vi "Process.vi"(8 "error in (no error)":errorcluster, 11 "Slave Test Runner In":refnum<class "Slave Test Runner.lvclass">) -> (0 "error out":errorcluster, 3 "Slave Test Runner Out":refnum<class "Slave Test Runner.lvclass">)   [LabVIEW 2020, in "Slave Test Runner.lvclass"]
uses:
  Slave Test Runner.lvclass
  C:/Users/anton/Documents/GitHub/LUnit/source/Application Framework/Process Classes/Process/Process.lvclass
  Application Framework/Process Classes/Process/Process.lvclass/Process.ctl
  Slave Test Runner.lvclass/Slave Test Runner.ctl
  Test Case/LUnit Test Case.lvclass
  Test Case/LUnit Test Case.lvclass/LUnit Test Case.ctl
  Result Classes/Method Result/Method Result.lvclass/Method Result.ctl
  Result Classes/Test Case Result/Test Case Result.lvclass/Test Case Result.ctl
  Result Collector/Result Collector.lvclass/Result Collector.ctl
  Result Collector/Result Collector.lvclass
  Private/SubVIs/Get all tests.vi
  Test Case/Community/SubVIs/Pre Test Case Reset.vi
  Private/SubVIs/Shuffle Test Methods.vi
  Private/SubVIs/Obtain Semaphores.vi
  Private/SubVIs/Write Test Case object to front panel control.vi
  Test Case/Community/SubVIs/Pre Method Reset.vi
  Test Case/Community/SubVIs/Get Test Method Result.vi
  Test Case/Community/SubVIs/Check For Errors.vi
  Private/SubVIs/Read Test Case object from front panel control.vi
  <vilib>/Utility/error.llb/Clear Errors.vi
  Private/SubVIs/Check Aborted.vi
  Private/SubVIs/Acquire Semaphore.vi
  Private/SubVIs/Release Semaphore.vi
  Private/SubVIs/Wait on VI to Execute.vi
  Test Case/Community/SubVIs/Set Test Method End Time.vi
  Private/SubVIs/Publish Method Result.vi
  Private/SubVIs/Publish Case Result.vi
  Test Case/Public/Accessors/Read Test Case Result.vi
  Application Framework/Process Classes/Process/Public/Accessors/Read Process Name.vi
  Test Case/Public/Accessors/Read Enabled Test Methods.vi
  Test Case/Private/SubVIs/Pre Allocate Method Results.vi
  Private/SubVIs/Shuffle Test Methods.vi/2fc74b80-6deb-4f17-a78e-34401938511c.vi
  Result Classes/Test Case Result/Public/Accessors/Read Method Results.vi
  Result Classes/Test Case Result/Community/Handle Error.vi
  Result Classes/Test Case Result/Community/Set Method End Time.vi
  Result Collector/Public/API/Collect Method Results.vi
  Result Collector/Public/API/Collect Case Result.vi
  Test Case/Private/SubVIs/Read Test Case Name.vi
  Result Classes/Test Case Result/Community/Preallocate Method Results.vi
  Result Classes/Method Result/Public/Read Status.vi
  Result Classes/Method Result/Community/Accessors/Generate Error.vi
  Result Classes/Method Result/Community/Accessors/Write Execution time.vi
  Result Classes/Method Result/Community/Accessors/Write Test Method Name.vi
  Result Classes/Method Result/Community/Accessors/Write Test Case.vi
  <vilib>/Utility/error.llb/Error Cluster From Error Code.vi
  <vilib>/Utility/LVClass/Get LV Class Name.vi
  <vilib>/Utility/semaphor.llb/Obtain Semaphore Reference.vi
  <vilib>/Utility/semaphor.llb/Acquire Semaphore.vi
  <vilib>/Utility/semaphor.llb/Release Semaphore.vi
  <vilib>/Utility/semaphor.llb/Release Semaphore Reference.vi
  Application Framework/Process Classes/Error Handler/Private/SubVIs/Get Error Queue Name.vi
  Result Classes/Test Case Result/Test Case Result.lvclass
  Result Classes/Method Result/Method Result.lvclass
  Application Framework/Process Classes/Process/Process.lvclass
  Application Framework/Process Classes/Error Handler/Error Handler.lvclass
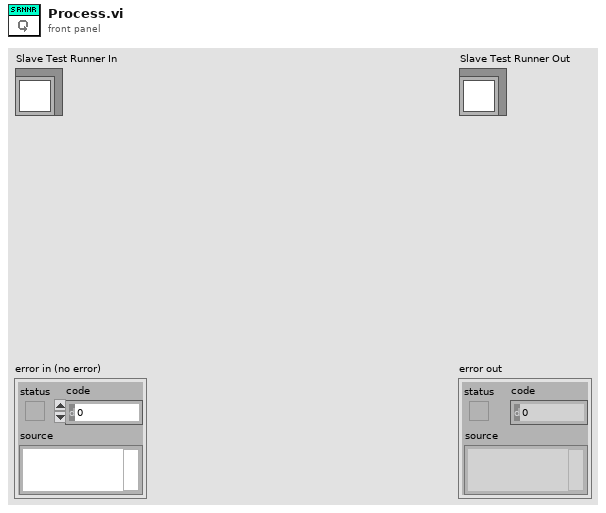
[diagram p1: front panel]
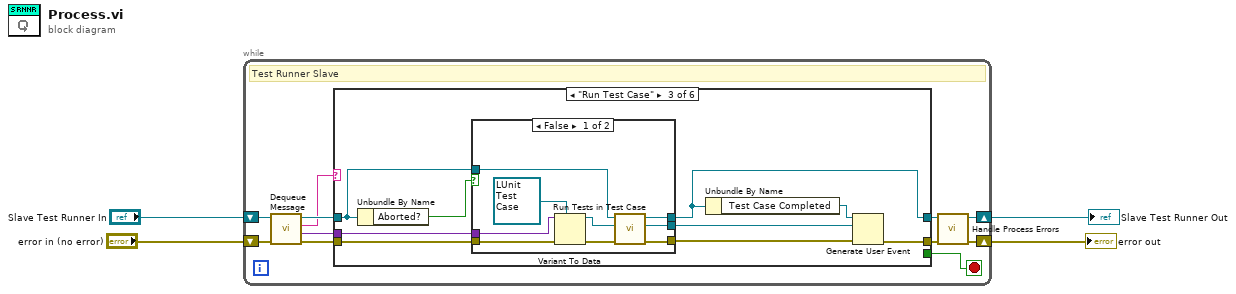
[diagram p0: block diagram]
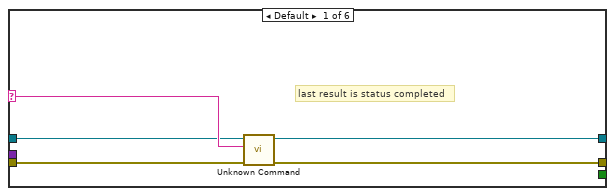
[diagram p2: hidden frame]
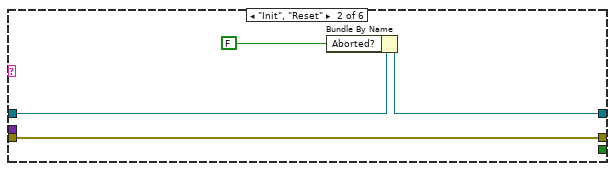
[diagram p3: hidden frame]
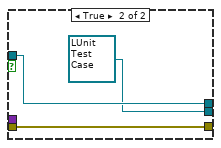
[diagram p4: hidden frame]
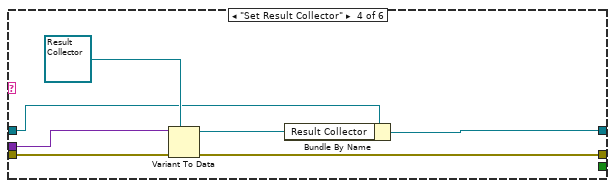
[diagram p5: hidden frame]
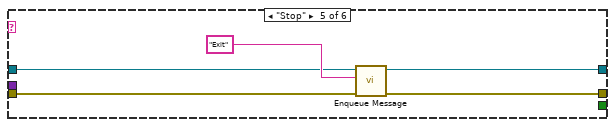
[diagram p6: hidden frame]
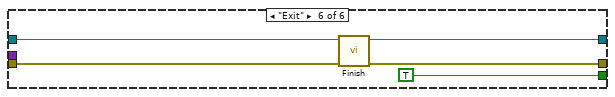
[diagram p7: hidden frame]
diagram:
  n1 = while {
    shift-right: [w5] -> w1
    shift-left: "error in (no error)" -> [w14]
    shift-right: [w7] -> w2
    shift-left: "Slave Test Runner In" -> [w15]
    stop <- w8 stop-if-true
    # "Test Runner Slave"
    n2 = call "Dequeue Message.vi"("error in (no error)"=w14, "Process In"=w15) -> ("error out"=w13:errorcluster, "Message Data"=w9:variant, "Message"=w10:string, "Process Out"=w11:refnum<class "Slave Test Runner.lvclass">)  [unwired: 6 in]
    n3 = case shown="\"Run Test Case\"" w10 {
      selector: w10 -> [w20 _ _ _ _ _]
      tunnel: [w17 w23 w31 w47 w54 w59] -> w6
      tunnel: w13 -> [w16 w23 w33 w52 w55 w58]
      tunnel: [w19 w22 w30 w46 w53 w60] -> w12
      tunnel: w11 -> [w18 w24 w29 w49 w56 w61]
      tunnel: w9 -> [_ _ w32 w51 _ _]
      tunnel: [_ _ _ _ _ TRUE] -> w8
      frame Default {
        # "last result is status completed"
        n4 = call "Unknown Command.vi"("error in (no error)"=w16, "String"=w20, "Process In"=w18) -> ("error out"=w17:errorcluster, "Process Out"=w19:refnum<class "Slave Test Runner.lvclass">)  [unwired: 7 in]
      }
      frame "Init", "Reset" {
        n5 = Bundle By Name(cluster=w24, "Aborted?"=FALSE) -> (w22:refnum<class "Slave Test Runner.lvclass">)
      }
      frame "Run Test Case" {
        n6 = Unbundle By Name(w29) -> ("Aborted?"=w25:bool)
        n7 = case shown="False" w25 {
          tunnel: w33 -> [w42 w44]
          tunnel: w32 -> [w41 _]
          tunnel: [w40 w45] -> w30
          tunnel: w29 -> [w39 w45]
          tunnel: [w35 w44] -> w27
          tunnel: [w34 refnum<class "LUnit Test Case.lvclass"> refnum ("Test Case out")] -> w26
          frame False {
            n8 = Variant To Data(error in=w42, type=refnum<class "LUnit Test Case.lvclass"> refnum ("Test Suite"), Variant=w41) -> (data=w36:refnum<class "LUnit Test Case.lvclass">, error out=w37:errorcluster)
            n9 = call "Run Tests in Test Case.vi"("error in (no error)"=w37, "Test Case"=w36, "Slave Test Runner In"=w39) -> ("error out"=w35:errorcluster, "Test Case out"=w34:refnum<class "LUnit Test Case.lvclass">, "Slave Test Runner Out"=w40:refnum<class "Slave Test Runner.lvclass">)  [unwired: 6 in]
          }
          frame True {
          }
        }
        n10 = Unbundle By Name(w30) -> ("Test Case Completed"=w28:refnum<user-event>)
        n11 = Generate User Event(user event=w28, event data cluster=w26, error in=w27) -> (error out=w31:errorcluster)  [unwired: 1 in, 1 out]
      }
      frame "Set Result Collector" {
        n12 = Variant To Data(error in=w52, type=refnum<class "Result Collector.lvclass"> refnum ("Test Report Generator.lvclass"), Variant=w51) -> (data=w48:refnum<class "Result Collector.lvclass">, error out=w47:errorcluster)
        n13 = Bundle By Name(cluster=w49, "Result Collector"=w48) -> (w46:refnum<class "Slave Test Runner.lvclass">)
      }
      frame "Stop" {
        n14 = call "Enqueue Message.vi"("error in (no error)"=w55, "Message"="Exit", "Process In"=w56) -> ("error out"=w54:errorcluster, "Process Out"=w53:refnum<class "Slave Test Runner.lvclass">)  [unwired: 7 in]
      }
      frame "Exit" {
        n15 = call "Finish.vi"("error in (no error)"=w58, "Process In"=w61) -> ("error out"=w59:errorcluster, "Process Out"=w60:refnum<class "Slave Test Runner.lvclass">)  [unwired: 8 in]
      }
    }
    n16 = call "Handle Process Errors.vi"("error in (no error)"=w6, "Process In"=w12) -> ("error out"=w5:errorcluster, "Process Out"=w7:refnum<class "Slave Test Runner.lvclass">)  [unwired: 8 in]
  }
  "error out" <- w1
  "Slave Test Runner Out" <- w2
